vi "Internal Sensors.vi"(8 "error in (no error)":errorcluster, 11 "output cluster":T1) -> (0 "error out":errorcluster)   [LabVIEW 2016]
uses:
  Queue Cluster TD.ctl
  Queue Attributes TD.ctl
  Queue Enum TD.ctl
  Internal data TD.ctl
  <vilib>/addons/zeromq/socket_type.ctl
  <vilib>/addons/zeromq/socket_options.ctl
  <vilib>/addons/zeromq/zeromq.lvlib
  <vilib>/addons/zeromq/zmq_context.lvclass
  <vilib>/addons/zeromq/zmq_socket.lvclass
panel:
  out "Intrinsic  Sensors":cluster{dbl, dbl, dbl}(graph)
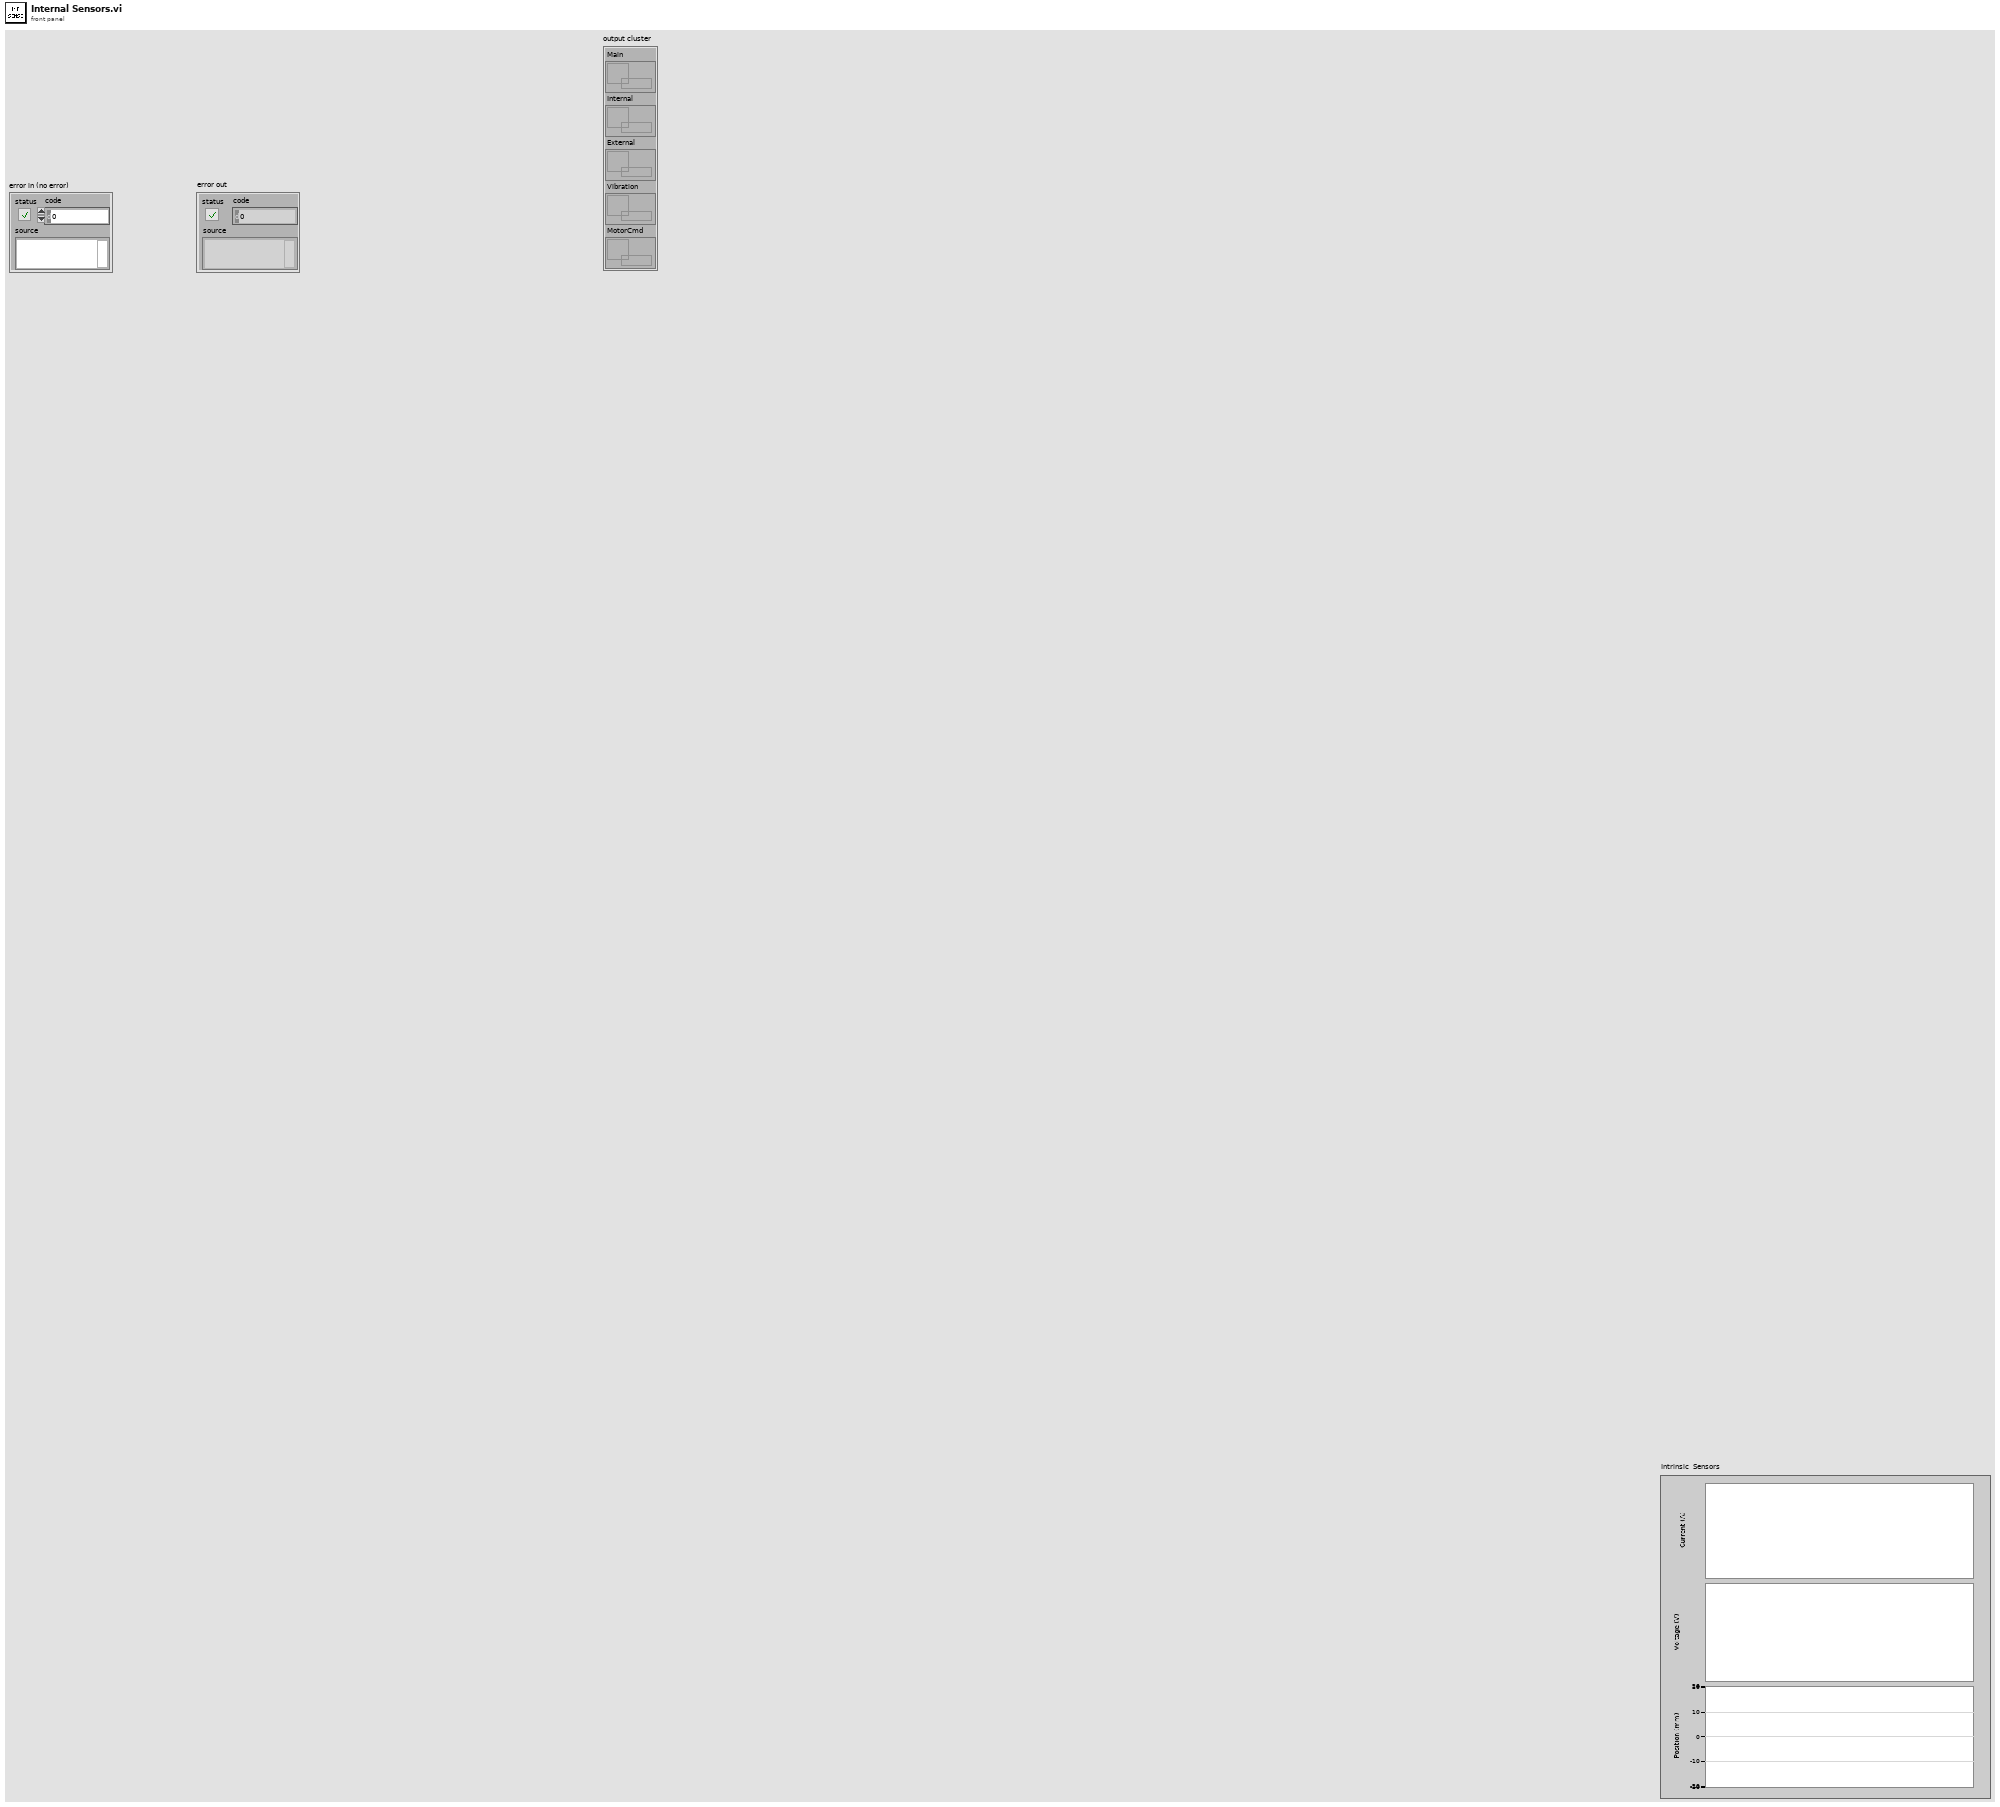
[diagram p1: front panel]
types:
  T1 = typedef "Queue Cluster TD.ctl" = cluster{"Main":refnum<queue>, "Internal":refnum<queue>, "External":refnum<queue>, "Vibration":refnum<queue>, "MotorCmd":refnum<queue>}
  T2 = typedef "Internal data TD.ctl" = cluster{"Current Data":string, "Voltage Data":string, "Position Data":string, "Connected?":bool, "Log File Refnum":refnum<file>, "Logging?":bool}
  T3 = typedef "Queue Attributes TD.ctl" = cluster{"State":T4, "String":string, "Boolean":bool, "Double":dbl, "U16":u16}
  T4 = typedef "Queue Enum TD.ctl" = enum16{"Stop", "Start", "Update D_HW", "Initialize", "Exit", "Read", "Write", "Plot", "Log", "Stop Log", "Start Log", "Wait"}
  T5 = typedef "zeromq.lvlib/socket_options.ctl" = enum8{"NONE", "ZMQ_HWM", "<2>", "ZMQ_SWAP", "ZMQ_AFFINITY", "ZMQ_IDENTITY", "ZMQ_SUBSCRIBE", "ZMQ_UNSUBSCRIBE", "ZMQ_RATE", "ZMQ_RECOVERY_IVL", "ZMQ_MCAST_LOOP", "ZMQ_SNDBUF", "ZMQ_RCVBUF", "ZMQ_RCVMORE", "ZMQ_FD", "ZMQ_EVENTS", "ZMQ_TYPE", "ZMQ_LINGER", "ZMQ_RECONNECT_IVL", "ZMQ_BACKLOG", "ZMQ_RECOVERY_IVL_MSEC", "ZMQ_RECONNECT_IVL_MAX", "ZMQ_MAXMSGSIZE", "ZMQ_SNDHWM", "ZMQ_RCVHWM", "ZMQ_MULTICAST_HOPS", "<26>", "ZMQ_RCVTIMEO", "ZMQ_SNDTIMEO", "<29>", "<30>", "ZMQ_IPV4ONLY", "ZMQ_LAST_ENDPOINT", "ZMQ_ROUTER_MANDATORY", "ZMQ_TCP_KEEPALIVE", "ZMQ_TCP_KEEPALIVE_CNT", "ZMQ_TCP_KEEPALIVE_IDLE", "ZMQ_TCP_KEEPALIVE_INTVL", "ZMQ_TCP_ACCEPT_FILTER", "ZMQ_DELAY_ATTACH_ON_CONNECT", "ZMQ_XPUB_VERBOSE"}
  T6 = typedef "zeromq.lvlib/socket_type.ctl" = enum8{"ZMQ_PAIR", "ZMQ_PUB", "ZMQ_SUB", "ZMQ_REQ", "ZMQ_REP", "ZMQ_DEALER", "ZMQ_ROUTER", "ZMQ_PULL", "ZMQ_PUSH", "ZMQ_XPUB", "ZMQ_XSUB"}
  T7 = enum16{"open", "replace", "create", "open or create", "replace or create", "replace or create with confirmation"}
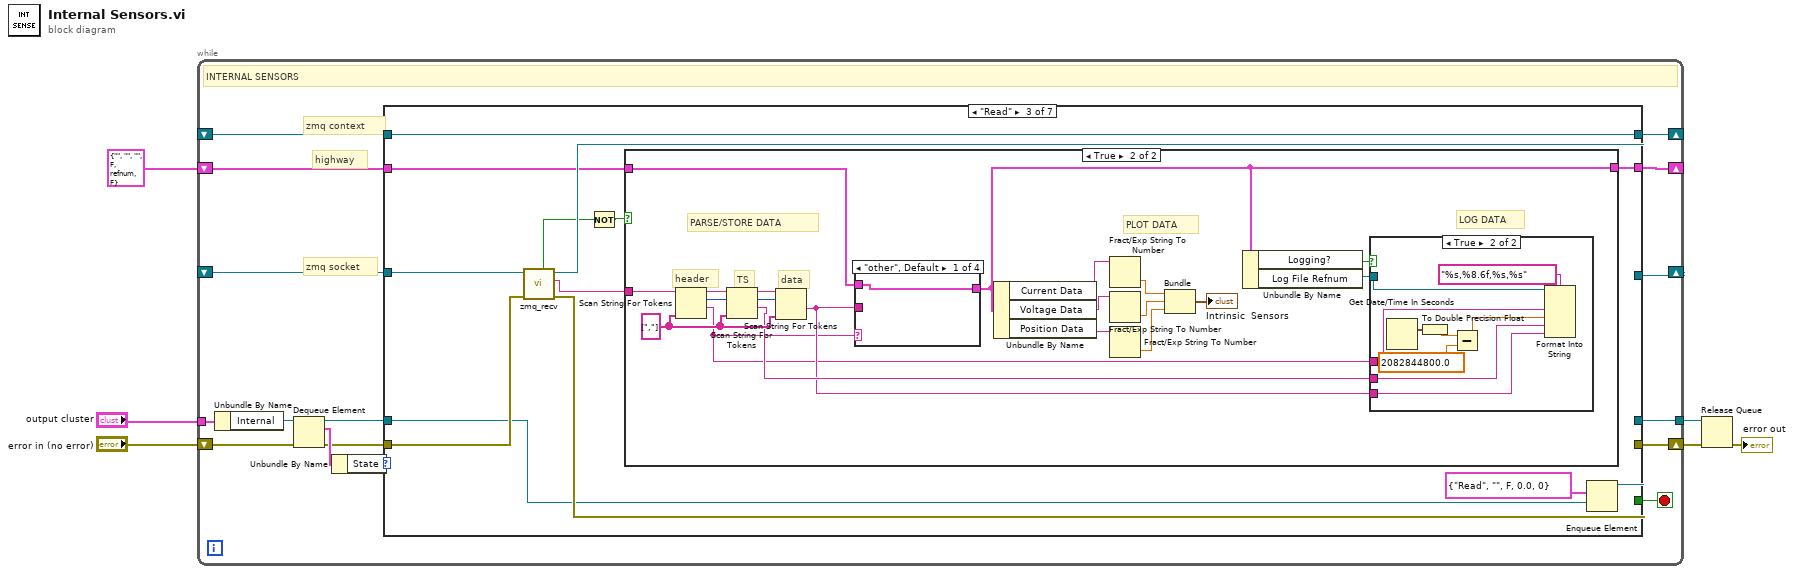
[diagram p0: block diagram]
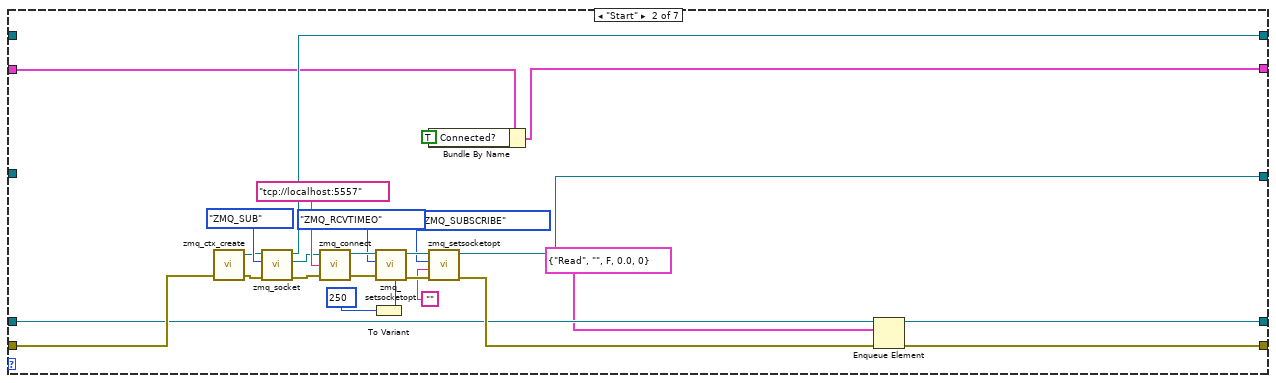
[diagram p3: hidden frame]
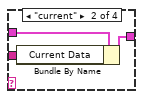
[diagram p6: hidden frame]
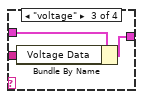
[diagram p7: hidden frame]
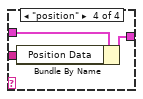
[diagram p8: hidden frame]
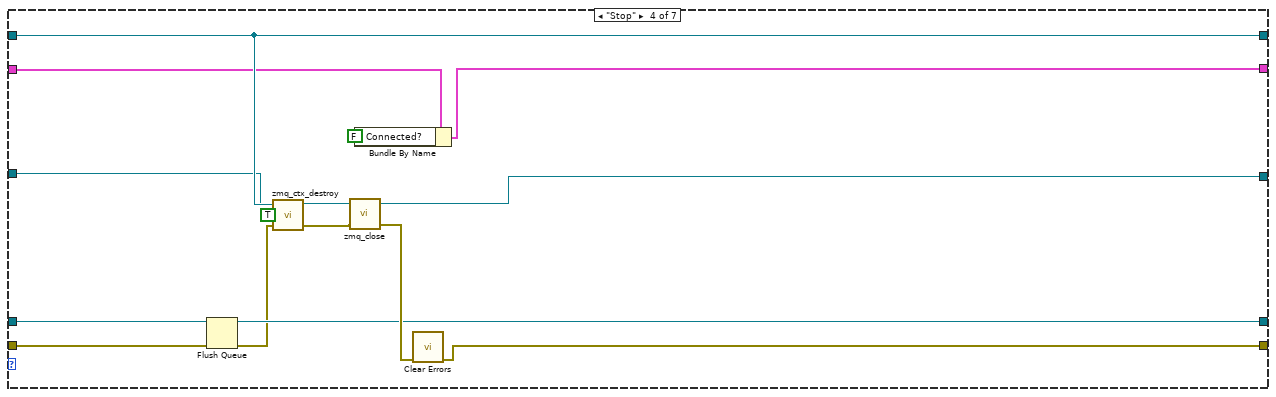
[diagram p9: hidden frame]
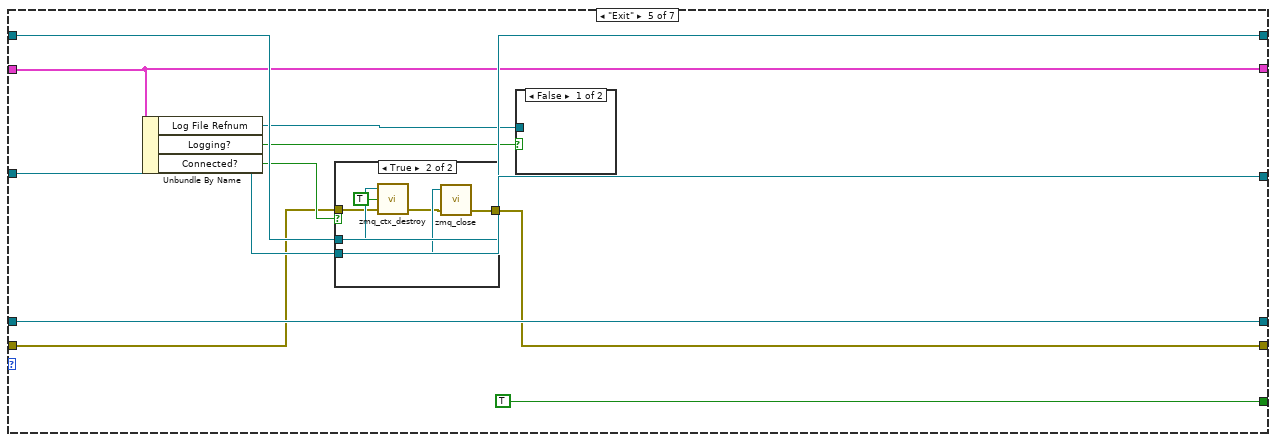
[diagram p10: hidden frame]
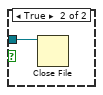
[diagram p11: hidden frame]
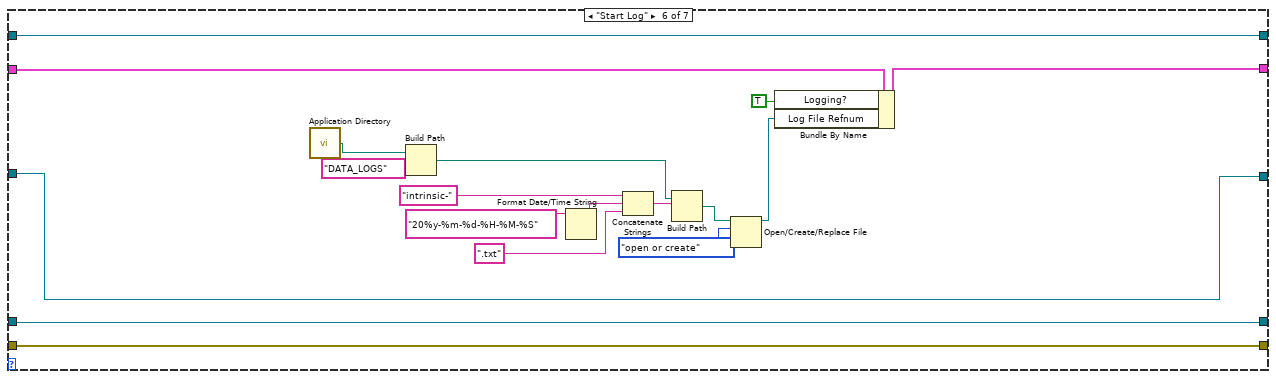
[diagram p13: hidden frame]
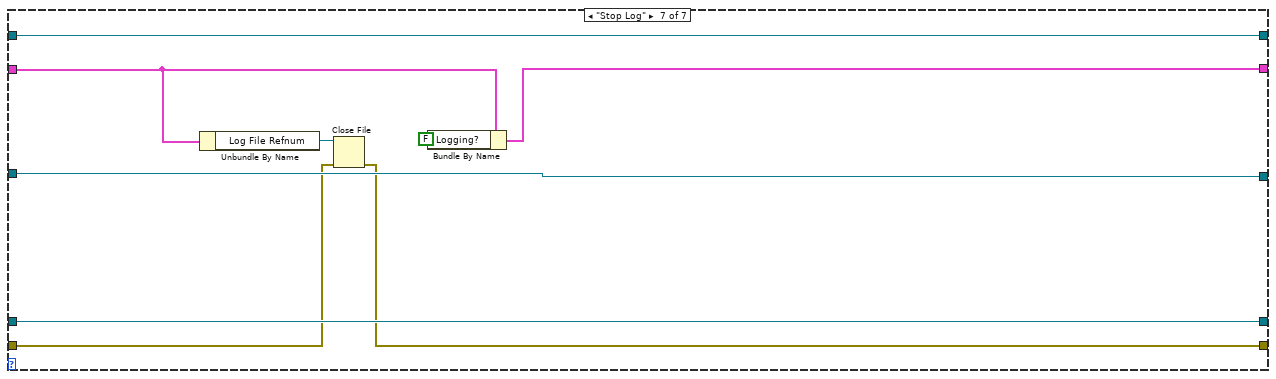
[diagram p14: hidden frame]
diagram:
  n1 = while {
    tunnel: "output cluster" -> [w22]
    tunnel: [w16] -> w5
    shift-right: [w15] -> w6
    shift-left: "error in (no error)" -> [w20]
    shift-right: [w12] -> _
    shift-left: _ -> [w11]
    shift-right: [w10] -> _
    shift-left: _ -> [w9]
    shift-right: [w7] -> _
    shift-left: T2 {"Current Data"="", "Voltage Data"="", "Position Data"="", "Connected?"=FALSE, "Log File Refnum"=refnum, "Logging?"=FALSE} ("Intrinsic Data Cluster TD") -> [w8]
    stop <- w13 stop-if-true
    # "highway"
    # "zmq socket"
    # "zmq context"
    # "INTERNAL SENSORS"
    n2 = Unbundle By Name(w22) -> ("Internal"=w21:refnum<queue>)
    n3 = Dequeue Element(queue=w21, error in (no error)=w20) -> (queue out=w17:refnum<queue>, element=w19:T3, error out=w18:errorcluster)  [unwired: 1 in, 1 out]
    n4 = Unbundle By Name(w19) -> ("State"=w14:T4)
    n5 = case shown="\"Read\"" w14 {
      tunnel: w18 -> [w26 w53 w65 w111 w121 w138 w161]
      tunnel: w17 -> [w27 w37 w58 w113 w129 w155 w164]
      tunnel: [w27 w36 w57 w112 w129 w155 w164] -> w16
      tunnel: [w26 w38 w60 w115 w120 w138 w160] -> w15
      tunnel: [_ _ _ _ TRUE _ _] -> w13
      tunnel: [w24 w34 w63 w118 w127 w139 w163] -> w12
      tunnel: w11 -> [w24 _ w64 w118 w127 w139 w163]
      tunnel: [w25 w33 w66 w119 w126 w154 w162] -> w10
      tunnel: w9 -> [w25 _ w66 w119 w126 w154 w162]
      tunnel: w8 -> [w23 w32 w62 w109 w123 w153 w157]
      tunnel: [w23 w31 w61 w108 w123 w152 w156] -> w7
      frame "Initialize", Default {
      }
      frame "Start" {
        n6 = call <vilib>:"zmq_ctx_create.vi"("error in"=w53) -> ("error out"=w45:errorcluster, "context out"=w44:refnum<class "zmq_context.lvclass">)  [unwired: 3 in]
        n7 = call <vilib>:"zmq_socket.vi"("error in"=w45, "socket type"=socket_type."ZMQ_SUB", "context in"=w44) -> ("error out"=w48:errorcluster, "socket out"=w47:refnum<class "zmq_socket.lvclass">, "context out"=w33:refnum<class "zmq_context.lvclass">)  [unwired: 2 in]
        n8 = call <vilib>:"zmq_connect.vi"("error in"=w48, "endpoint"="tcp://localhost:5557", "socket in"=w47) -> ("error out"=w52:errorcluster, "socket out"=w51:refnum<class "zmq_socket.lvclass">)  [unwired: 1 in]
        n9 = To Variant(anything=250) -> (Variant=w28:variant)
        n10 = call <vilib>:"zmq_setsocketopt.vi"("error in"=w52, "value"=w28, "option"=socket_options."ZMQ_RCVTIMEO", "socket in"=w51) -> ("error out"=w42:errorcluster, "socket out"=w43:refnum<class "zmq_socket.lvclass">)  [unwired: 2 in]
        n11 = Bundle By Name(cluster=w32, "Connected?"=TRUE) -> (w31:T2)
        n12 = call <vilib>:"zmq_setsocketopt.vi"("error in"=w42, "value"="", "option"=socket_options."ZMQ_SUBSCRIBE", "socket in"=w43) -> ("error out"=w39:errorcluster, "socket out"=w34:refnum<class "zmq_socket.lvclass">)  [unwired: 2 in]
        n13 = Enqueue Element(queue=w37, element=T3 {"State"=enum."Read", "String"="", "Boolean"=FALSE, "Double"=0.0, "U16"=0}, error in (no error)=w39) -> (queue out=w36:refnum<queue>, error out=w38:errorcluster)  [unwired: 1 in, 1 out]
      }
      frame "Read" {
        n14 = call <vilib>:"zmq_recv.vi"("error in"=w65, "socket in"=w64) -> ("error out"=w60:errorcluster, "data"=w56:string, "socket out"=w63:refnum<class "zmq_socket.lvclass">, "timeout?"=w54:bool)  [unwired: 3 in, 1 out]
        n15 = Not(x=w54) -> (.not. x?=w55:bool)
        n16 = case shown="True" w55 {
          tunnel: w62 -> [w67 w76]
          tunnel: w56 -> [_ w71]
          tunnel: [w67 w69] -> w61
          frame False {
          }
          frame True {
            w87 = string[] [","]
            # "LOG DATA"
            # "PLOT DATA"
            # "PARSE/STORE DATA"
            # "data"
            # "TS"
            # "header"
            n17 = Scan String For Tokens(6:w87, 9:w71) -> (1:w77:string, 2:w85:i32, 3:w86:string)  [unwired: 4 in, 1 out]
            n18 = Scan String For Tokens(6:w87, 8:w85, 9:w86) -> (1:w83:string, 2:w70:i32, 3:w84:string)  [unwired: 3 in, 1 out]
            n19 = Scan String For Tokens(6:w87, 8:w70, 9:w84) -> (1:w82:string)  [unwired: 3 in, 3 out]
            n20 = case shown="\"other\", Default" w77 {
              tunnel: w82 -> [_ w100 w103 w106]
              tunnel: [w97 w99 w102 w105] -> w69
              tunnel: w76 -> [w97 w98 w101 w104]
              frame "other", Default {
              }
              frame "current" {
                n21 = Bundle By Name(cluster=w98, "Current Data"=w100) -> (w99:T2)
              }
              frame "voltage" {
                n22 = Bundle By Name(cluster=w101, "Voltage Data"=w103) -> (w102:T2)
              }
              frame "position" {
                n23 = Bundle By Name(cluster=w104, "Position Data"=w106) -> (w105:T2)
              }
            }
            n24 = Unbundle By Name(w69) -> ("Current Data"=w73:string, "Voltage Data"=w75:string, "Position Data"=w74:string)
            n25 = Fract/Exp String To Number(string=w73) -> (number=w81:dbl)  [unwired: 3 in, 1 out]
            n26 = Fract/Exp String To Number(string=w75) -> (number=w80:dbl)  [unwired: 3 in, 1 out]
            n27 = Fract/Exp String To Number(string=w74) -> (number=w79:dbl)  [unwired: 3 in, 1 out]
            n28 = Bundle(w81, w80, w79) -> (→"Intrinsic  Sensors":cluster{dbl, dbl, dbl})  [unwired: 1 in]
            n29 = Unbundle By Name(w69) -> ("Logging?"=w72:bool, "Log File Refnum"=w78:refnum<file>)
            n30 = case shown="True" w72 {
              tunnel: w77 -> [_ w88]
              tunnel: w83 -> [_ w91]
              tunnel: w82 -> [_ w90]
              tunnel: w78 -> [_ w89]
              frame False {
              }
              frame True {
                n31 = Get Date/Time In Seconds() -> (seconds since 1Jan1904=w95:timestamp)
                n32 = To Double Precision Float(number=w95) -> (double precision float=w94:dbl)
                n33 = Subtract(x=w94, y=2082844800.0 ("Epoch Delta (s)")) -> (x-y=w92:dbl)
                n34 = Format Into String(format string="%s,%8.6f,%s,%s", initial string=w89, w88, w92, w91, w90) -> ()  [unwired: 1 in, 2 out]
              }
            }
          }
        }
        n35 = Enqueue Element(queue=w58, element=T3 {"State"=enum."Read", "String"="", "Boolean"=FALSE, "Double"=0.0, "U16"=0}) -> (queue out=w57:refnum<queue>)  [unwired: 2 in, 2 out]
      }
      frame "Stop" {
        n36 = Flush Queue(queue=w113, error in (no error)=w111) -> (queue out=w112:refnum<queue>, error out=w110:errorcluster)  [unwired: 1 out]
        n37 = call <vilib>:"zmq_ctx_destroy.vi"("error in"=w110, "reap? (F)"=TRUE, "context in"=w119) -> ("error out"=w117:errorcluster)  [unwired: 2 in]
        n38 = call <vilib>:"zmq_close.vi"("error in"=w117, "socket"=w118) -> ("error out"=w116:errorcluster)  [unwired: 3 in]
        n39 = Bundle By Name(cluster=w109, "Connected?"=FALSE) -> (w108:T2)
        n40 = call <vilib>:"Clear Errors.vi"("error in (no error)"=w116) -> ("error out"=w115:errorcluster)  [unwired: 5 in, 1 out]
      }
      frame "Exit" {
        n41 = Unbundle By Name(w123) -> ("Log File Refnum"=w122:refnum<file>, "Logging?"=w124:bool, "Connected?"=w125:bool)
        n42 = case shown="True" w125 {
          tunnel: w127 -> [_ w137]
          tunnel: w126 -> [_ w136]
          tunnel: w121 -> [w131 w135]
          tunnel: [w131 w133] -> w120
          frame False {
          }
          frame True {
            n43 = call <vilib>:"zmq_ctx_destroy.vi"("error in"=w135, "reap? (F)"=TRUE, "context in"=w136) -> ("error out"=w134:errorcluster)  [unwired: 2 in]
            n44 = call <vilib>:"zmq_close.vi"("error in"=w134, "socket"=w137) -> ("error out"=w133:errorcluster)  [unwired: 3 in]
          }
        }
        n45 = case shown="False" w124 {
          tunnel: w122 -> [_ w130]
          frame False {
          }
          frame True {
            n46 = Close File(refnum=w130) -> ()  [unwired: 1 in, 2 out]
          }
        }
      }
      frame "Start Log" {
        n47 = call <vilib>:"Application Directory.vi"() -> ("Application Directory"=w144:path)
        n48 = Build Path(base path=w144, name or relative path="DATA_LOGS") -> (appended path=w145:path)
        n49 = Format Date/Time String(time format string (%c)="20%y-%m-%d-%H-%M-%S") -> (date/time string=w147:string)  [unwired: 2 in]
        n50 = Concatenate Strings("intrinsic-" ("Data type"), w147, ".txt") -> (w150:string)
        n51 = Build Path(base path=w145, name or relative path=w150) -> (appended path=w151:path)
        n52 = Open/Create/Replace File(file path (use dialog)=w151, operation (0:open)=T7."open or create") -> (refnum out=w141:refnum<file>)  [unwired: 4 in, 2 out]
        n53 = Bundle By Name(cluster=w153, "Logging?"=TRUE, "Log File Refnum"=w141) -> (w152:T2)
      }
      frame "Stop Log" {
        n54 = Unbundle By Name(w157) -> ("Log File Refnum"=w159:refnum<file>)
        n55 = Close File(refnum=w159, error in=w161) -> (error out=w160:errorcluster)  [unwired: 1 out]
        n56 = Bundle By Name(cluster=w157, "Logging?"=FALSE) -> (w156:T2)
      }
    }
  }
  n57 = Release Queue(queue=w5, error in (no error)=w6) -> (error out=→"error out":errorcluster)  [unwired: 1 in, 2 out]
